vi "Environement Datalogger.vi"() -> ()   [LabVIEW 2011]
uses:
  Classes/IP Connection/IP Connection.lvclass
  Classes/Temperature IR Bricklet/Temperature IR Bricklet.lvclass
  Classes/Humidity Bricklet/Humidity Bricklet.lvclass
  Classes/Ambient Light Bricklet/Ambient Light Bricklet.lvclass
panel:
  out "Multicolumn Listbox":i32(listbox)
  out "Waveform Chart":T1(graph)
  in  "Stop Button":bool
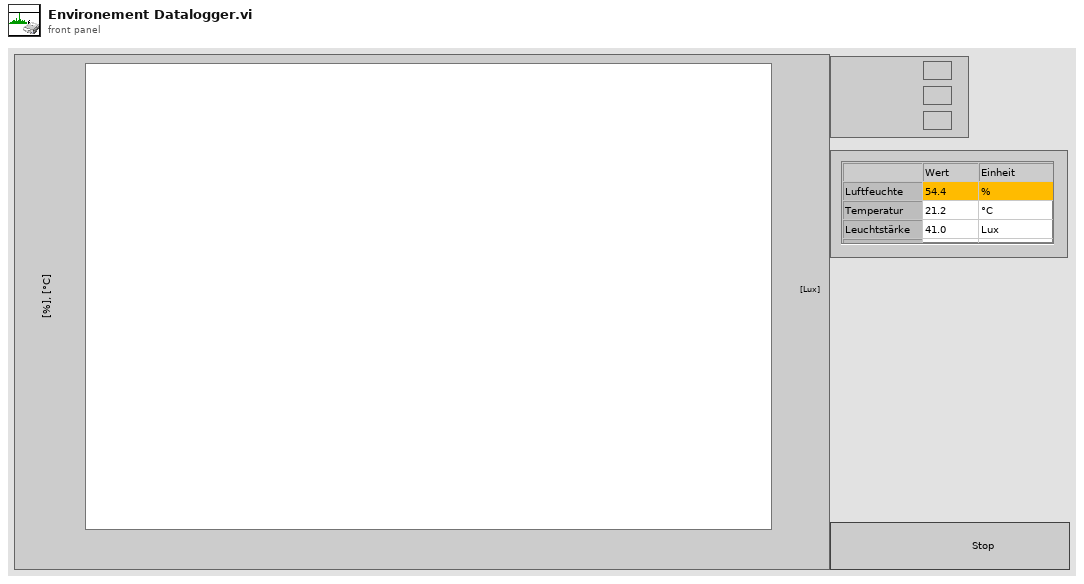
[diagram p1: front panel]
types:
  T1 = cluster{"Value scaled":dbl, "Value scaled":dbl, "Value scaled":dbl}
  T2 = cluster{"Value scaled":dbl, "Value scaled":dbl, "Value scaled":dbl}[]
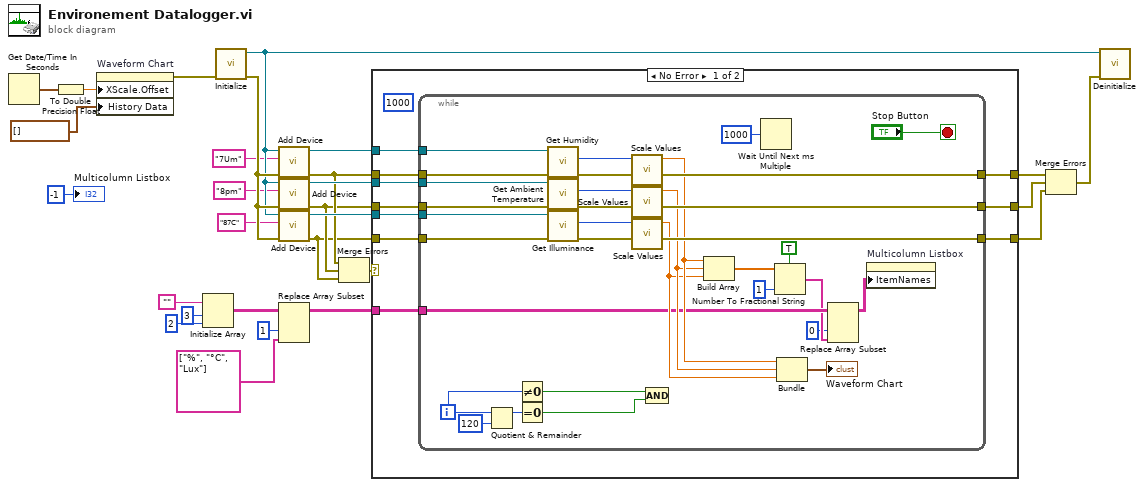
[diagram p0: block diagram]
diagram:
  n1 = Get Date/Time In Seconds() -> (seconds since 1Jan1904=w14:timestamp)
  n2 = To Double Precision Float(number=w14) -> (double precision float=w13:dbl)
  n3 = property on="Waveform Chart" class="WFChart (strict)"("XScale.Offset"=w13, "History Data"=T2 []) -> (error out=w15:errorcluster)  [unwired: 2 in, 1 out]
  n4 = Initialize Array("", 3 ("dimension size"), 2 ("dimension size")) -> (w3:string[][])
  n5 = call "Initialize.vi"("error in (no error)"=w15) -> ("error out"=w28:errorcluster, "IP Connection out"=w24:refnum<class "IP Connection.lvclass">)  [unwired: 9 in]
  n6 = call "Add Device.vi"("Error In"=w28, "Device UID"="7Um", "IP Connection"=w24) -> ("Error Out"=w22:errorcluster, "Humidity Bricklet"=w27:refnum<class "Humidity Bricklet.lvclass">)  [unwired: 7 in]
  n7 = call "Add Device.vi"("Error In"=w28, "Device UID"="8pm", "IP Connection"=w24) -> ("Error Out"=w21:errorcluster, "Ambient Light Bricklet"=w26:refnum<class "Temperature IR Bricklet.lvclass">)  [unwired: 7 in]
  n8 = call "Add Device.vi"("Error In"=w28, "Device UID"="87C", "IP Connection"=w24) -> ("Error Out"=w20:errorcluster, "Ambient Light Bricklet"=w25:refnum<class "Ambient Light Bricklet.lvclass">)  [unwired: 7 in]
  n9 = Replace Array Subset(array=w3, new element=string[] ["%", "°C", "Lux"], index (col)=1 ("disabled index (col)")) -> (w2:string[][])  [unwired: 1 in]
  n10 = Merge Errors(w22, w21, w20) -> (w19:errorcluster)
  n11 = case shown="No Error" w19 {
    tunnel: w22 -> [w38 w71]
    tunnel: w27 -> [w37 _]
    tunnel: w26 -> [w36 _]
    tunnel: w21 -> [w35 w70]
    tunnel: w25 -> [w34 _]
    tunnel: w20 -> [w33 w69]
    tunnel: [w32 w71] -> w18
    tunnel: [w31 w70] -> w17
    tunnel: [w30 w69] -> w16
    tunnel: w2 -> [w29 _]
    frame No Error {
      (unwired) 1000
      n12 = while {
        tunnel: w38 -> [w68]
        tunnel: w37 -> [w67]
        tunnel: w36 -> [w66]
        tunnel: w35 -> [w65]
        tunnel: w34 -> [w64]
        tunnel: w33 -> [w63]
        tunnel: [w62] -> w32
        tunnel: [w61] -> w31
        tunnel: [w60] -> w30
        tunnel: w29 -> [w48]
        i -> [w57]
        stop <- "Stop Button" stop-if-true
        n13 = Quotient & Remainder(x=w57, y=120) -> (x-y*floor(x/y)=w58:i32)  [unwired: 1 out]
        n14 = Not Equal To 0?(x=w57) -> (x != 0?=w56:bool)
        n15 = Equal To 0?(x=w58) -> (x = 0?=w55:bool)
        n16 = call "Get Humidity.vi"("error in (no error)"=w68, "Humidity Bricklet in"=w67) -> ("error out"=w62:errorcluster, "Humidity"=w54:u16)  [unwired: 7 in, 1 out]
        n17 = call "Get Ambient Temperature.vi"("error in (no error)"=w65, "Temperature IR Bricklet in"=w66) -> ("error out"=w61:errorcluster, "Ambient Temperature"=w53:i16)  [unwired: 7 in, 1 out]
        n18 = call "Get Illuminance.vi"("error in (no error)"=w63, "Ambient Light Bricklet in"=w64) -> ("error out"=w60:errorcluster, "Illuminance"=w52:u16)  [unwired: 7 in, 1 out]
        n19 = call "Scale Values.vi"("Value"=w54) -> ("Value scaled"=w51:dbl)  [unwired: 10 in]
        n20 = call "Scale Values.vi"("Value"=w53) -> ("Value scaled"=w50:dbl)  [unwired: 10 in]
        n21 = call "Scale Values.vi"("Value"=w52) -> ("Value scaled"=w49:dbl)  [unwired: 10 in]
        n22 = Compound Arithmetic op=AND(w56, w55) -> ()  [unwired: 1 out]
        n23 = Build Array(w51, w50, w49) -> (w45:dbl[])
        n24 = Wait Until Next ms Multiple(millisecond multiple=u32 1000) -> ()  [unwired: 1 out]
        n25 = Number To Fractional String(use system decimal point (T)=TRUE, number=w45, precision (6)=i16 1) -> (F-format string=w42:string[])  [unwired: 1 in]
        n26 = Bundle("Value scaled"=w51, "Value scaled"=w50, "Value scaled"=w49) -> (→"Waveform Chart":T1)  [unwired: 1 in]
        n27 = Replace Array Subset(array=w48, new element=w42, index (col)=0 ("disabled index (col)")) -> (w41:string[][])  [unwired: 1 in]
        n28 = property on="Multicolumn Listbox" class="MCListbox (strict)"("ItemNames"=w41) -> ()  [unwired: 2 in, 2 out]
      }
    }
    frame Error {
    }
  }
  n29 = Merge Errors(w18, w17, w16) -> (w23:errorcluster)
  n30 = call "Deinitialize.vi"("error in (no error)"=w23, "IP Connection in"=w24) -> ()  [unwired: 9 in, 1 out]
  "Multicolumn Listbox" <- -1 ("Multicolumn Listbox")
